vi "cDAQ Kill Digitizing Process.vi"(8 "error in":errorcluster, 11 "cdaq session in":T1={"mclk [Hz]"=12800000.0, "ADC task"="", "mclk reference"="", "fs [Hz]"=50000.0, "queue adc cmd"=refnum, "queue adc data"=refnum, "adc proc ref"=refnum, "channels"=[], "last channels"=[], "timeout"=timestamp(0 s since 1904-01-01), "N"=1000} {"last channels"."Channel id" min=0 step=1; "channels"."Channel id" min=0 step=1}) -> (0 "error out":errorcluster, 3 "cdaq session out":T1={"mclk [Hz]"=12800000.0, "ADC task"="", "mclk reference"="", "fs [Hz]"=50000.0, "queue adc cmd"=refnum, "queue adc data"=refnum, "adc proc ref"=refnum, "channels"=[], "last channels"=[], "timeout"=timestamp(0 s since 1904-01-01), "N"=1000} {"last channels"."Channel id" min=0 step=1; "channels"."Channel id" min=0 step=1})   [LabVIEW 2013]
uses:
  cDAQ Session.ctl
  low_level_old/cdaq_anal_adc_command.ctl
  low_level_old/cdaq_anal_adc_data.ctl
  cDAQ Virtual Channel.ctl
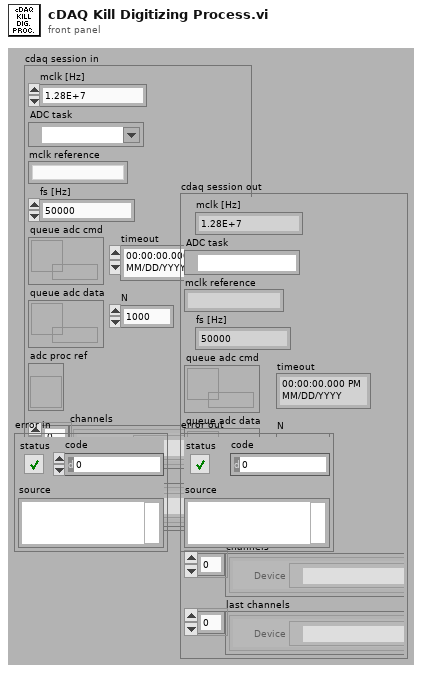
[diagram p1: front panel]
types:
  T1 = typedef "cDAQ Session.ctl" = cluster{"mclk [Hz]":dbl, "ADC task":refnum<k21>, "mclk reference":string, "fs [Hz]":dbl, "queue adc cmd":refnum<queue>, "queue adc data":refnum<queue>, "adc proc ref":refnum<vi>, "channels":T2[], "last channels":T2[], "timeout":timestamp, "N":i32}
  T2 = typedef "cDAQ Virtual Channel.ctl" = cluster{"Device":tag, "Channel id":i32, "btn clr":bool, "btn up":bool, "btn down":bool}
  T3 = typedef "cdaq_anal_adc_command.ctl" = cluster{"sample to get":i32, "stop":bool, "abort":bool}
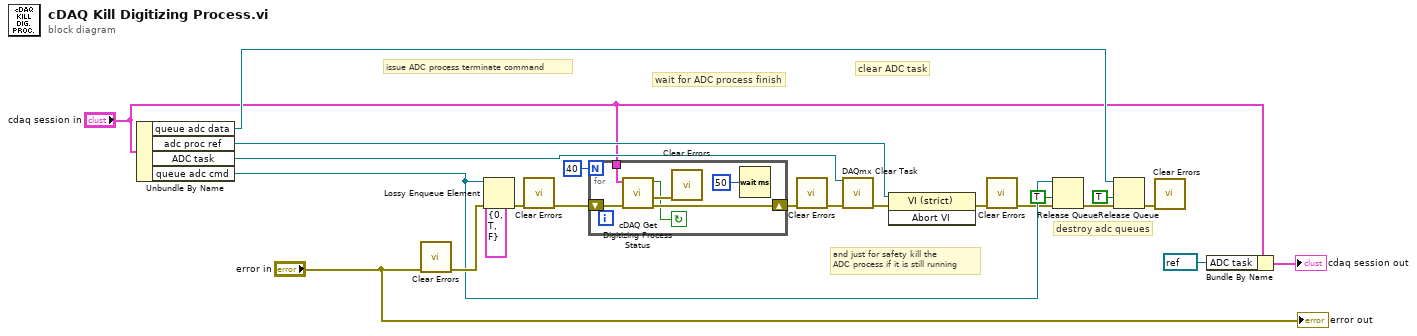
[diagram p0: block diagram]
diagram:
  # "destroy adc queues"
  # "and just for safety kill the\nADC process if it is still running"
  # "clear ADC task"
  # "wait for ADC process finish"
  # "issue ADC process terminate command"
  n1 = Unbundle By Name("cdaq session in") -> ("queue adc data"=w7:refnum<queue>, "adc proc ref"=w12:refnum<vi>, "ADC task"=w14:refnum<k21>, "queue adc cmd"=w10:refnum<queue>)
  n2 = call <vilib>:"Clear Errors.vi"("error in (no error)"="error in") -> ("error out"=w13:errorcluster)  [unwired: 6 in]
  n3 = Lossy Enqueue Element(queue=w10, element=T3 {"sample to get"=0, "stop"=TRUE, "abort"=FALSE}, error in (no error)=w13) -> (error out=w19:errorcluster)  [unwired: 3 out]
  n4 = call <vilib>:"Clear Errors.vi"("error in (no error)"=w19) -> ("error out"=w18:errorcluster)  [unwired: 6 in]
  n5 = for {
    N: 40 -> [_]
    shift-right: [w27] -> w16
    shift-left: w18 -> [w28]
    tunnel: "cdaq session in" -> [w23]
    stop <- w25 continue-if-true
    n6 = call "cDAQ Get Digitizing Process Status.vi"("error in"=w28, "cdaq session"=w23) -> ("error out"=w27:errorcluster, "sweep error out"=w26:errorcluster, "is running"=w25:bool)  [unwired: 7 in]
    n7 = call <vilib>:"Clear Errors.vi"("error in (no error)"=w26) -> ()  [unwired: 6 in, 1 out]
    n8 = Wait (ms)(milliseconds to wait=u32 50) -> ()  [unwired: 1 out]
  }
  n9 = call <vilib>:"Clear Errors.vi"("error in (no error)"=w16) -> ("error out"=w15:errorcluster)  [unwired: 6 in]
  n10 = call <vilib>:"DAQmx Clear Task.vi"("task in"=w14, "error in"=w15) -> ("error out"=w11:errorcluster)  [unwired: 13 in]
  n11 = invoke class="VI (strict)" method="Abort VI"(reference=w12, error in=w11) -> (error out=w5:errorcluster)  [unwired: 1 in, 2 out]
  n12 = call <vilib>:"Clear Errors.vi"("error in (no error)"=w5) -> ("error out"=w4:errorcluster)  [unwired: 6 in]
  n13 = Release Queue(queue=w10, force destroy? (F)=TRUE, error in (no error)=w4) -> (error out=w8:errorcluster)  [unwired: 2 out]
  n14 = Release Queue(queue=w7, force destroy? (F)=TRUE, error in (no error)=w8) -> (error out=w3:errorcluster)  [unwired: 2 out]
  n15 = call <vilib>:"Clear Errors.vi"("error in (no error)"=w3) -> ()  [unwired: 6 in, 1 out]
  n16 = Bundle By Name(cluster="cdaq session in", "ADC task"=refnum<k21> refnum) -> (→"cdaq session out":T1)
  "error out" <- "error in"
